vi "DuplicateLabels.vi"(9 "String":string, 10 "Numeric":dbl, 11 "Numeric":dbl) -> ()   [LabVIEW 2011]
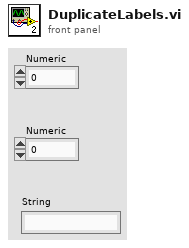
[diagram p1: front panel]
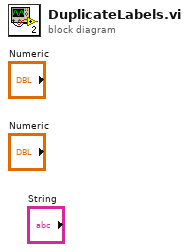
[diagram p0: block diagram]
diagram:
